vi "car_tcp.vi"() -> ()   [LabVIEW 2022 SP3]
uses:
  Control 1.ctl
  Control 2.ctl
  chicken.ctl
  plus_one.ctl
  game_over.ctl
  Control 4.ctl
  tree_control.ctl
panel:
  out "Boolean 12":T1
  in  "chicken":T2
  in  "tree 2":T3
  in  "tree":T3
  in  "tree 5":T3
  in  "tree 4":T3
  out "TOP":i16
  out "SCORE":i16
  in  "stop":bool
  in  "tree 3":T3
  out "Boolean 11":T4
  out "grass 5":T5
  out "grass 4":T5
  out "grass 3":T5
  out "grass 2":T5
  out "grass 1":T5
  out "easy?":bool
  in  "HARD":bool
  in  "EASY":bool
  out "car_x":i16
  out "Boolean 10":T6
  in  "v 10":dbl
  in  "v 9":dbl
  out "Boolean 9":T7
  in  "v 8":dbl
  out "Boolean 8":T6
  in  "v 7":dbl
  out "Boolean 7":T7
  out "Boolean 6":T6
  in  "v 6":dbl
  in  "v 5":dbl
  out "Boolean 5":T7
  in  "v 4":dbl
  out "Boolean 4":T6
  in  "v 3":dbl
  out "Boolean 3":T7
  in  "v 2":dbl
  in  "v":dbl
  out "Boolean 2":T6
  out "Boolean":T7
  # "SCORE"
  # "TOP"
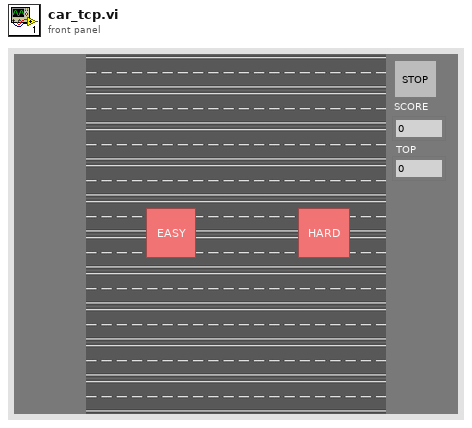
[diagram p1: front panel]
types:
  T1 = typedef "game_over.ctl" = bool
  T2 = typedef "chicken.ctl" = bool
  T3 = typedef "tree_control.ctl" = bool
  T4 = typedef "plus_one.ctl" = bool
  T5 = typedef "Control 4.ctl" = bool
  T6 = typedef "Control 2.ctl" = bool
  T7 = typedef "Control 1.ctl" = bool
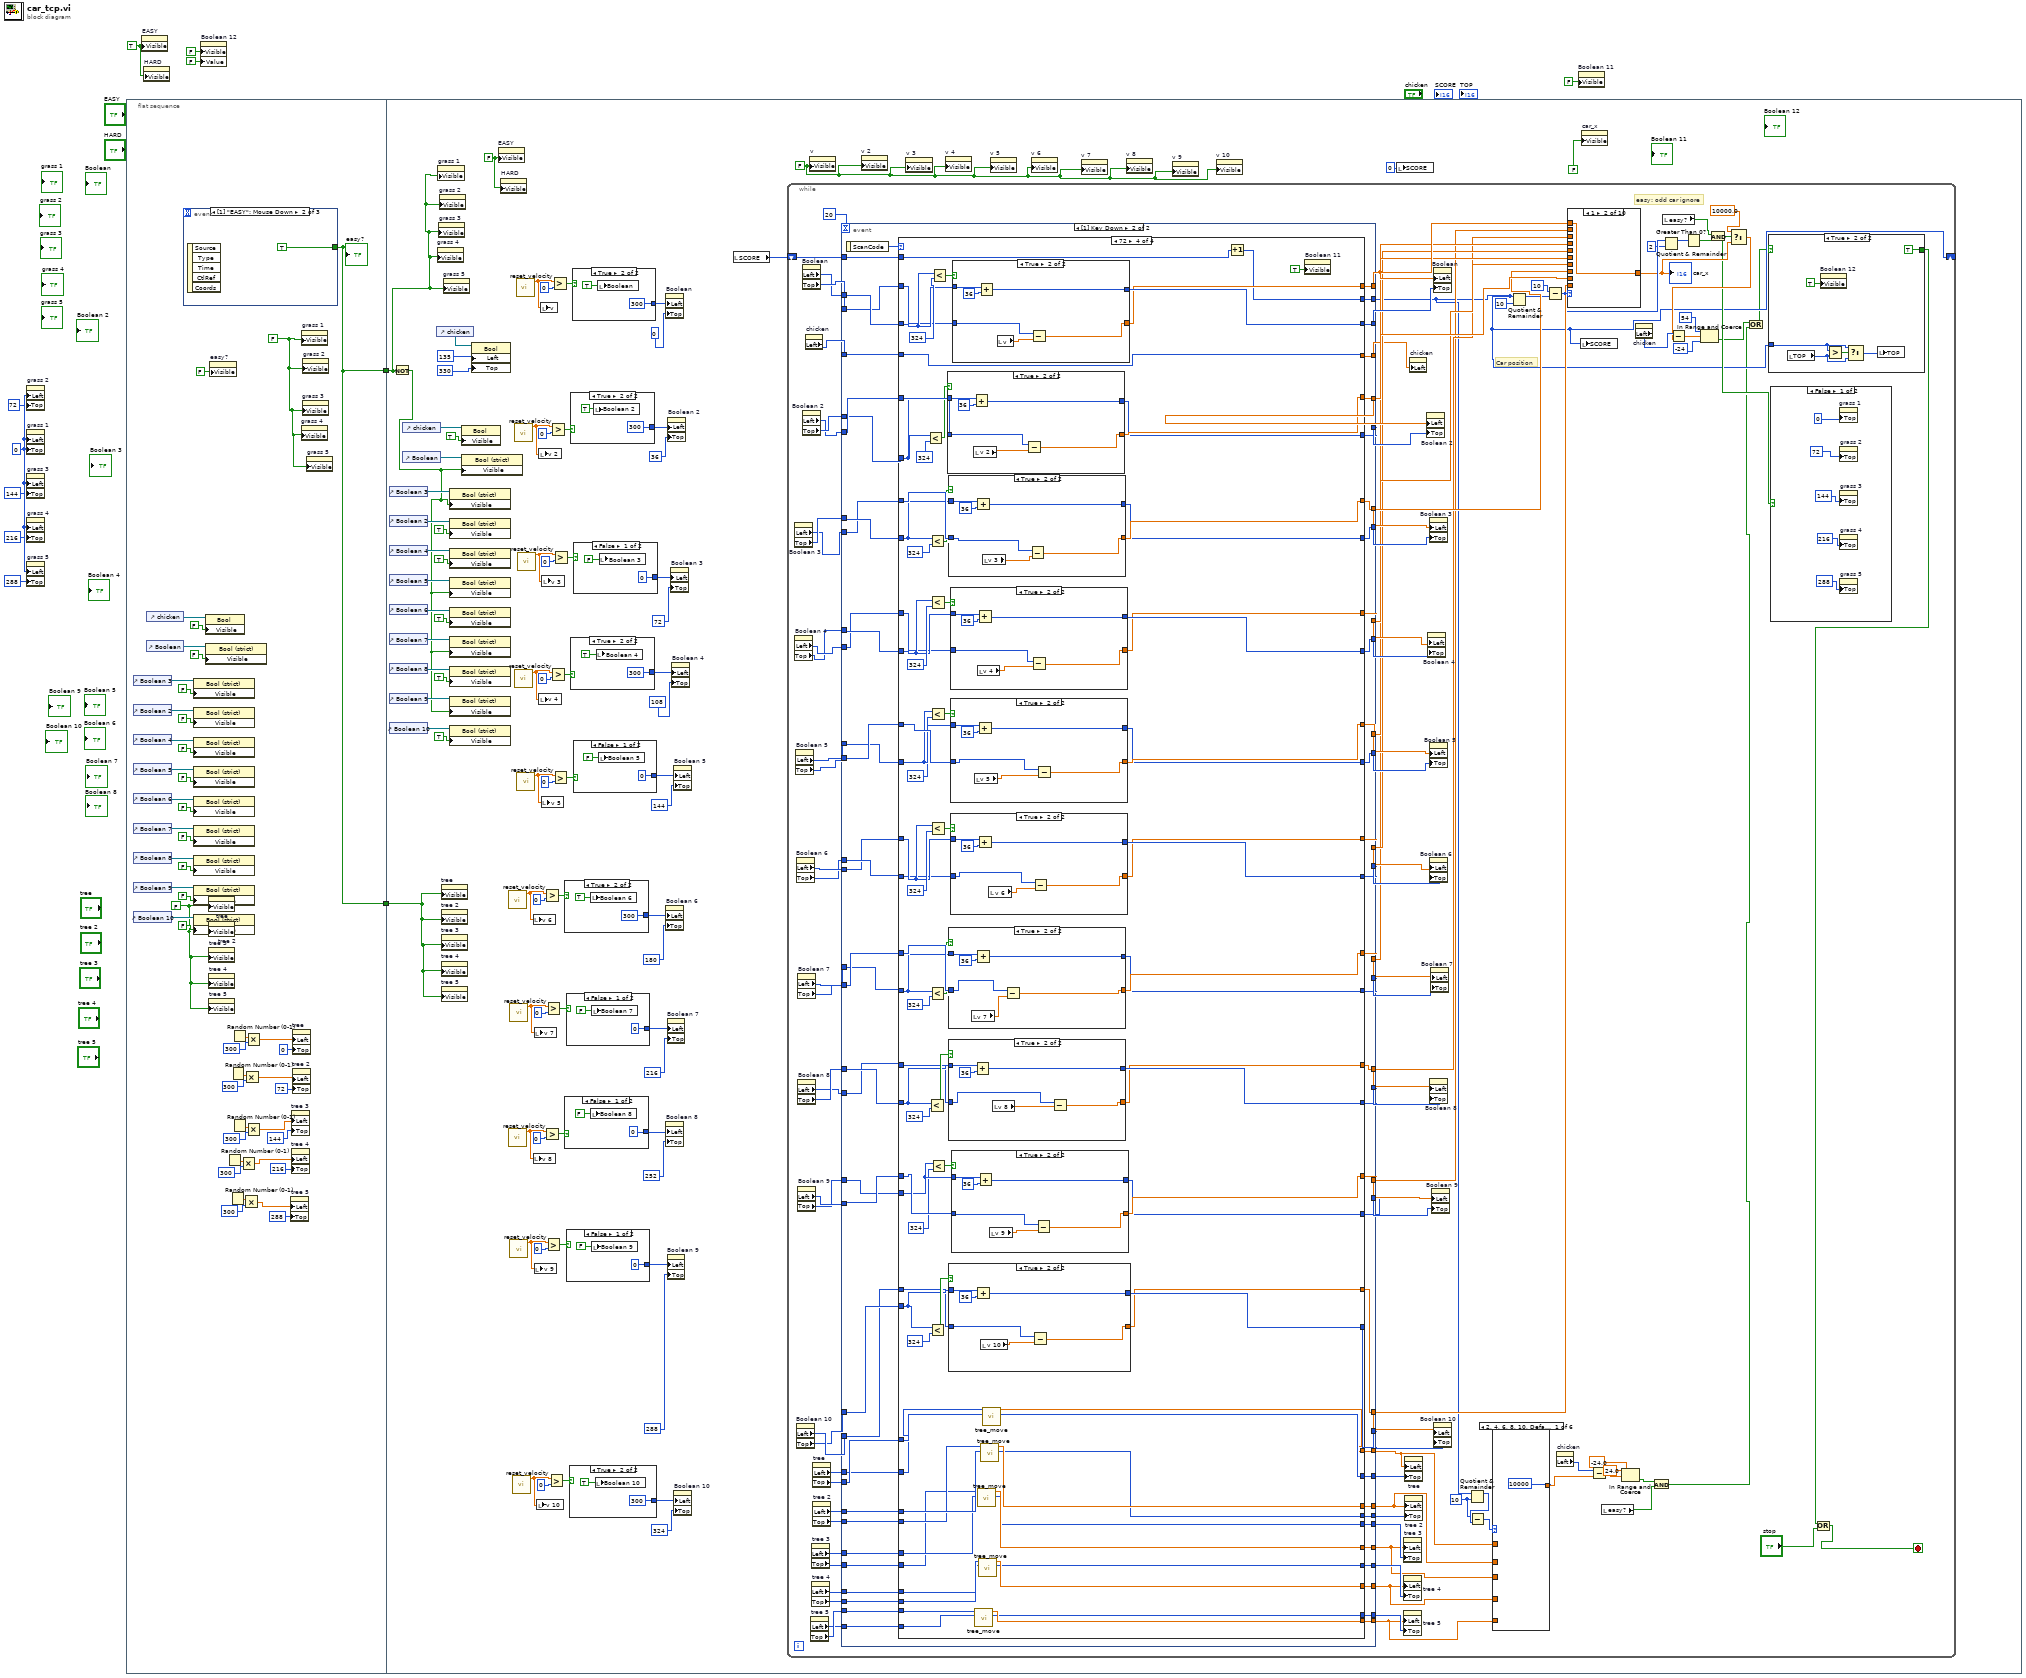
[diagram p0: block diagram]
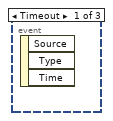
[diagram p2: hidden frame]
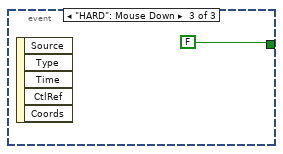
[diagram p3: hidden frame]
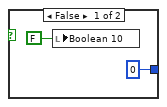
[diagram p4: hidden frame]
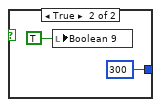
[diagram p5: hidden frame]
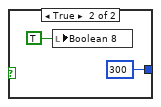
[diagram p6: hidden frame]
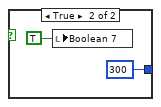
[diagram p7: hidden frame]
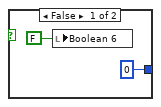
[diagram p8: hidden frame]
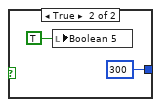
[diagram p9: hidden frame]
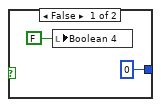
[diagram p10: hidden frame]
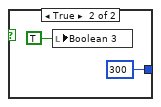
[diagram p11: hidden frame]
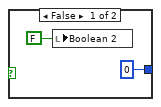
[diagram p12: hidden frame]
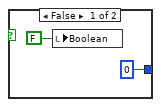
[diagram p13: hidden frame]
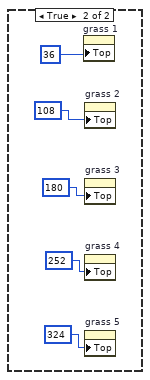
[diagram p19: hidden frame]
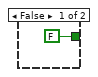
[diagram p20: hidden frame]
diagram:
  w6 = 0
  w8 = TRUE ("Visible")
  n1 = property on="grass 2" class="Bool"("Left"=w6, "Top"=72) -> ()  [unwired: 2 in, 2 out]
  n2 = property on="grass 1" class="Bool"("Left"=w6, "Top"=w6) -> ()  [unwired: 2 in, 2 out]
  n3 = property on="grass 3" class="Bool"("Left"=w6, "Top"=144) -> ()  [unwired: 2 in, 2 out]
  n4 = property on="grass 4" class="Bool"("Left"=w6, "Top"=216) -> ()  [unwired: 2 in, 2 out]
  n5 = property on="grass 5" class="Bool"("Left"=w6, "Top"=288) -> ()  [unwired: 2 in, 2 out]
  n6 = flat-sequence {
    tunnel: [w32] -> w7
    tunnel: [w32] -> w1
    tunnel: w7 -> [w62]
    tunnel: w1 -> [w60]
    frame #0 {
      w33 = FALSE
      w34 = FALSE ("Visible")
      n7 = control-ref of="Boolean 3"() -> (w44:refnum<vi>)
      n8 = control-ref of="Boolean 2"() -> (w43:refnum<vi>)
      n9 = control-ref of="Boolean 4"() -> (w42:refnum<vi>)
      n10 = control-ref of="Boolean 5"() -> (w41:refnum<vi>)
      n11 = control-ref of="Boolean 6"() -> (w40:refnum<vi>)
      n12 = control-ref of="Boolean 7"() -> (w39:refnum<vi>)
      n13 = control-ref of="Boolean 8"() -> (w38:refnum<vi>)
      n14 = control-ref of="Boolean 9"() -> (w37:refnum<vi>)
      n15 = control-ref of="Boolean 10"() -> (w35:refnum<vi>)
      n16 = control-ref of="chicken"() -> (w56:refnum<vi>)
      n17 = control-ref of="Boolean"() -> (w45:refnum<vi>)
      n18 = event shown="[1] \"EASY\": Mouse Down" {
        selector: _ -> [_ _ _]
        dyn-events: _ -> [_ _ _]
        timeout: _ -> [_ _ _]
        tunnel: [_ TRUE FALSE] -> w32
        event Timeout {
          n19 = event-data() -> ()  [unwired: 1 in, 3 out]
        }
        event "EASY": Mouse Down {
          n20 = event-data() -> ()  [unwired: 1 in, 5 out]
        }
        event "HARD": Mouse Down {
          n21 = event-data() -> ()  [unwired: 1 in, 5 out]
        }
      }
      "easy?" <- w32
      n22 = property class="Bool (strict)"(reference=w44, "Visible"=FALSE) -> ()  [unwired: 1 in, 2 out]
      n23 = property class="Bool (strict)"(reference=w43, "Visible"=FALSE) -> ()  [unwired: 1 in, 2 out]
      n24 = property class="Bool (strict)"(reference=w42, "Visible"=FALSE) -> ()  [unwired: 1 in, 2 out]
      n25 = property class="Bool (strict)"(reference=w41, "Visible"=FALSE) -> ()  [unwired: 1 in, 2 out]
      n26 = property class="Bool (strict)"(reference=w40, "Visible"=FALSE) -> ()  [unwired: 1 in, 2 out]
      n27 = property class="Bool (strict)"(reference=w39, "Visible"=FALSE) -> ()  [unwired: 1 in, 2 out]
      n28 = property class="Bool (strict)"(reference=w38, "Visible"=FALSE) -> ()  [unwired: 1 in, 2 out]
      n29 = property class="Bool (strict)"(reference=w37, "Visible"=FALSE) -> ()  [unwired: 1 in, 2 out]
      n30 = property class="Bool (strict)"(reference=w35, "Visible"=FALSE) -> ()  [unwired: 1 in, 2 out]
      n31 = property class="Bool"(reference=w56, "Visible"=FALSE) -> ()  [unwired: 1 in, 2 out]
      n32 = property class="Bool (strict)"(reference=w45, "Visible"=FALSE) -> ()  [unwired: 1 in, 2 out]
      n33 = property on="tree" class="Bool"("Visible"=w33) -> ()  [unwired: 2 in, 2 out]
      n34 = property on="tree 2" class="Bool"("Visible"=w33) -> ()  [unwired: 2 in, 2 out]
      n35 = property on="tree 3" class="Bool"("Visible"=w33) -> ()  [unwired: 2 in, 2 out]
      n36 = property on="tree 4" class="Bool"("Visible"=w33) -> ()  [unwired: 2 in, 2 out]
      n37 = property on="tree 5" class="Bool"("Visible"=w33) -> ()  [unwired: 2 in, 2 out]
      n38 = property on="easy?" class="Bool (strict)"("Visible"=FALSE) -> ()  [unwired: 2 in, 2 out]
      n39 = Random Number (0-1)() -> (number: 0 to 1=w23:dbl)
      n40 = Random Number (0-1)() -> (number: 0 to 1=w22:dbl)
      n41 = Random Number (0-1)() -> (number: 0 to 1=w27:dbl)
      n42 = Random Number (0-1)() -> (number: 0 to 1=w31:dbl)
      n43 = Random Number (0-1)() -> (number: 0 to 1=w26:dbl)
      n44 = Multiply(x=w23, y=300) -> (x*y=w18:dbl)
      n45 = Multiply(x=w22, y=300) -> (x*y=w17:dbl)
      n46 = Multiply(x=w27, y=300) -> (x*y=w20:dbl)
      n47 = Multiply(x=w31, y=300) -> (x*y=w29:dbl)
      n48 = Multiply(x=w26, y=300) -> (x*y=w19:dbl)
      n49 = property on="tree 5" class="Bool"("Left"=w17, "Top"=288 ("Position:Top")) -> ()  [unwired: 2 in, 2 out]
      n50 = property on="tree 3" class="Bool"("Left"=w19, "Top"=144 ("Position:Top")) -> ()  [unwired: 2 in, 2 out]
      n51 = property on="tree 4" class="Bool"("Left"=w18, "Top"=216 ("Position:Top")) -> ()  [unwired: 2 in, 2 out]
      n52 = property on="tree" class="Bool"("Left"=w29, "Top"=0 ("Position:Top")) -> ()  [unwired: 2 in, 2 out]
      n53 = property on="tree 2" class="Bool"("Left"=w20, "Top"=72 ("Position:Top")) -> ()  [unwired: 2 in, 2 out]
      n54 = property on="grass 4" class="Bool"("Visible"=w34) -> ()  [unwired: 2 in, 2 out]
      n55 = property on="grass 1" class="Bool"("Visible"=w34) -> ()  [unwired: 2 in, 2 out]
      n56 = property on="grass 3" class="Bool"("Visible"=w34) -> ()  [unwired: 2 in, 2 out]
      n57 = property on="grass 2" class="Bool"("Visible"=w34) -> ()  [unwired: 2 in, 2 out]
      n58 = property on="grass 5" class="Bool"("Visible"=w34) -> ()  [unwired: 2 in, 2 out]
    }
    frame #1 {
      w81 = FALSE ("Visible")
      w96 = FALSE ("Visible")
      n59 = control-ref of="Boolean 3"() -> (w71:refnum<vi>)
      n60 = control-ref of="Boolean 2"() -> (w72:refnum<vi>)
      n61 = control-ref of="Boolean 4"() -> (w73:refnum<vi>)
      n62 = control-ref of="Boolean 5"() -> (w74:refnum<vi>)
      n63 = control-ref of="Boolean 6"() -> (w75:refnum<vi>)
      n64 = control-ref of="Boolean 7"() -> (w76:refnum<vi>)
      n65 = control-ref of="Boolean 8"() -> (w77:refnum<vi>)
      n66 = control-ref of="Boolean 9"() -> (w78:refnum<vi>)
      n67 = control-ref of="Boolean 10"() -> (w80:refnum<vi>)
      n68 = Not(x=w62) -> (.not. x?=w63:bool)
      n69 = control-ref of="chicken"() -> (w64:refnum<vi>)
      n70 = control-ref of="Boolean"() -> (w70:refnum<vi>)
      n71 = control-ref of="chicken"() -> (w86:refnum<vi>)
      n72 = property on="grass 4" class="Bool"("Visible"=w62) -> ()  [unwired: 2 in, 2 out]
      n73 = property on="grass 1" class="Bool"("Visible"=w62) -> ()  [unwired: 2 in, 2 out]
      n74 = property on="grass 3" class="Bool"("Visible"=w62) -> ()  [unwired: 2 in, 2 out]
      n75 = property on="grass 2" class="Bool"("Visible"=w62) -> ()  [unwired: 2 in, 2 out]
      n76 = property on="tree" class="Bool"("Visible"=w60) -> ()  [unwired: 2 in, 2 out]
      n77 = property on="tree 2" class="Bool"("Visible"=w60) -> ()  [unwired: 2 in, 2 out]
      n78 = property on="tree 3" class="Bool"("Visible"=w60) -> ()  [unwired: 2 in, 2 out]
      n79 = property on="tree 4" class="Bool"("Visible"=w60) -> ()  [unwired: 2 in, 2 out]
      n80 = property on="tree 5" class="Bool"("Visible"=w60) -> ()  [unwired: 2 in, 2 out]
      n81 = property on="grass 5" class="Bool"("Visible"=w62) -> ()  [unwired: 2 in, 2 out]
      n82 = property class="Bool (strict)"(reference=w71, "Visible"=w63) -> ()  [unwired: 1 in, 2 out]
      n83 = property class="Bool (strict)"(reference=w72, "Visible"=TRUE) -> ()  [unwired: 1 in, 2 out]
      n84 = property class="Bool (strict)"(reference=w73, "Visible"=TRUE) -> ()  [unwired: 1 in, 2 out]
      n85 = property class="Bool (strict)"(reference=w74, "Visible"=w63) -> ()  [unwired: 1 in, 2 out]
      n86 = property class="Bool (strict)"(reference=w75, "Visible"=TRUE) -> ()  [unwired: 1 in, 2 out]
      n87 = property class="Bool (strict)"(reference=w76, "Visible"=w63) -> ()  [unwired: 1 in, 2 out]
      n88 = property class="Bool (strict)"(reference=w77, "Visible"=TRUE) -> ()  [unwired: 1 in, 2 out]
      n89 = property class="Bool (strict)"(reference=w78, "Visible"=w63) -> ()  [unwired: 1 in, 2 out]
      n90 = property class="Bool (strict)"(reference=w80, "Visible"=TRUE) -> ()  [unwired: 1 in, 2 out]
      n91 = property class="Bool"(reference=w64, "Visible"=TRUE) -> ()  [unwired: 1 in, 2 out]
      n92 = property class="Bool (strict)"(reference=w70, "Visible"=w63) -> ()  [unwired: 1 in, 2 out]
      n93 = property on="Property Node" class="Bool"(reference=w86, "Left"=135 ("Position:Left"), "Top"=330 ("Position:Top")) -> ()  [unwired: 1 in, 2 out]
      n94 = property on="EASY" class="Bool"("Visible"=w81) -> ()  [unwired: 2 in, 2 out]
      n95 = property on="HARD" class="Bool"("Visible"=w81) -> ()  [unwired: 2 in, 2 out]
      n96 = call "reset_velocity.vi"() -> ("Numeric"=w91:dbl)  [unwired: 11 in]
      n97 = call "reset_velocity.vi"() -> ("Numeric"=w89:dbl)  [unwired: 11 in]
      n98 = call "reset_velocity.vi"() -> ("Numeric"=w90:dbl)  [unwired: 11 in]
      n99 = call "reset_velocity.vi"() -> ("Numeric"=w88:dbl)  [unwired: 11 in]
      n100 = call "reset_velocity.vi"() -> ("Numeric"=w87:dbl)  [unwired: 11 in]
      n101 = call "reset_velocity.vi"() -> ("Numeric"=w95:dbl)  [unwired: 11 in]
      n102 = call "reset_velocity.vi"() -> ("Numeric"=w93:dbl)  [unwired: 11 in]
      n103 = call "reset_velocity.vi"() -> ("Numeric"=w137:dbl)  [unwired: 11 in]
      n104 = call "reset_velocity.vi"() -> ("Numeric"=w92:dbl)  [unwired: 11 in]
      n105 = call "reset_velocity.vi"() -> ("Numeric"=w94:dbl)  [unwired: 11 in]
      n106 = local write "v 6"(w91) -> ()
      n107 = local write "v 8"(w89) -> ()
      n108 = local write "v 7"(w90) -> ()
      n109 = local write "v 9"(w88) -> ()
      n110 = local write "v 10"(w87) -> ()
      n111 = local write "v 2"(w95) -> ()
      n112 = local write "v 4"(w93) -> ()
      n113 = local write "v"(w137) -> ()
      n114 = local write "v 5"(w92) -> ()
      n115 = local write "v 3"(w94) -> ()
      n116 = Greater?(x=w91, y=0) -> (0:w116:bool)
      n117 = Greater?(x=w89, y=0) -> (0:w108:bool)
      n118 = Greater?(x=w90, y=0) -> (0:w111:bool)
      n119 = Greater?(x=w88, y=0) -> (0:w103:bool)
      n120 = Greater?(x=w87, y=0) -> (0:w100:bool)
      n121 = Greater?(x=w95, y=0) -> (0:w132:bool)
      n122 = Greater?(x=w93, y=0) -> (0:w124:bool)
      n123 = Greater?(x=w137, y=0) -> (0:w135:bool)
      n124 = Greater?(x=w92, y=0) -> (0:w119:bool)
      n125 = Greater?(x=w94, y=0) -> (0:w127:bool)
      n126 = case shown="True" w116 {
        tunnel: [0 300] -> w114
        frame False {
          n127 = local write "Boolean 6"(FALSE) -> ()
        }
        frame True {
          n128 = local write "Boolean 6"(TRUE) -> ()
        }
      }
      n129 = case shown="False" w108 {
        tunnel: [0 300] -> w106
        frame False {
          n130 = local write "Boolean 8"(FALSE) -> ()
        }
        frame True {
          n131 = local write "Boolean 8"(TRUE) -> ()
        }
      }
      n132 = case shown="False" w111 {
        tunnel: [0 300] -> w110
        frame False {
          n133 = local write "Boolean 7"(FALSE) -> ()
        }
        frame True {
          n134 = local write "Boolean 7"(TRUE) -> ()
        }
      }
      n135 = case shown="False" w103 {
        tunnel: [0 300] -> w102
        frame False {
          n136 = local write "Boolean 9"(FALSE) -> ()
        }
        frame True {
          n137 = local write "Boolean 9"(TRUE) -> ()
        }
      }
      n138 = case shown="True" w100 {
        tunnel: [0 300] -> w98
        frame False {
          n139 = local write "Boolean 10"(FALSE) -> ()
        }
        frame True {
          n140 = local write "Boolean 10"(TRUE) -> ()
        }
      }
      n141 = case shown="True" w132 {
        tunnel: [0 300] -> w130
        frame False {
          n142 = local write "Boolean 2"(FALSE) -> ()
        }
        frame True {
          n143 = local write "Boolean 2"(TRUE) -> ()
        }
      }
      n144 = case shown="True" w124 {
        tunnel: [0 300] -> w122
        frame False {
          n145 = local write "Boolean 4"(FALSE) -> ()
        }
        frame True {
          n146 = local write "Boolean 4"(TRUE) -> ()
        }
      }
      n147 = case shown="True" w135 {
        tunnel: [0 300] -> w134
        frame False {
          n148 = local write "Boolean"(FALSE) -> ()
        }
        frame True {
          n149 = local write "Boolean"(TRUE) -> ()
        }
      }
      n150 = case shown="False" w119 {
        tunnel: [0 300] -> w118
        frame False {
          n151 = local write "Boolean 5"(FALSE) -> ()
        }
        frame True {
          n152 = local write "Boolean 5"(TRUE) -> ()
        }
      }
      n153 = case shown="False" w127 {
        tunnel: [0 300] -> w125
        frame False {
          n154 = local write "Boolean 3"(FALSE) -> ()
        }
        frame True {
          n155 = local write "Boolean 3"(TRUE) -> ()
        }
      }
      n156 = property on="Boolean" class="Bool (strict)"("Left"=w134, "Top"=0) -> ()  [unwired: 2 in, 2 out]
      n157 = property on="Boolean 6" class="Bool (strict)"("Left"=w114, "Top"=180) -> ()  [unwired: 2 in, 2 out]
      n158 = property on="Boolean 8" class="Bool (strict)"("Left"=w106, "Top"=252) -> ()  [unwired: 2 in, 2 out]
      n159 = property on="Boolean 7" class="Bool (strict)"("Left"=w110, "Top"=216) -> ()  [unwired: 2 in, 2 out]
      n160 = property on="Boolean 9" class="Bool (strict)"("Left"=w102, "Top"=288) -> ()  [unwired: 2 in, 2 out]
      n161 = property on="Boolean 2" class="Bool (strict)"("Left"=w130, "Top"=36) -> ()  [unwired: 2 in, 2 out]
      n162 = property on="Boolean 3" class="Bool (strict)"("Left"=w125, "Top"=72) -> ()  [unwired: 2 in, 2 out]
      n163 = property on="Boolean 4" class="Bool (strict)"("Left"=w122, "Top"=108) -> ()  [unwired: 2 in, 2 out]
      n164 = property on="Boolean 5" class="Bool (strict)"("Left"=w118, "Top"=144) -> ()  [unwired: 2 in, 2 out]
      n165 = property on="Boolean 10" class="Bool (strict)"("Left"=w98, "Top"=324) -> ()  [unwired: 2 in, 2 out]
      n166 = local read "SCORE"() -> (w61:i16)
      n167 = while {
        shift-right: [w196] -> _
        shift-left: w61 -> [w212]
        stop <- w230 stop-if-true
        w194 = i16 10 ("y")
        # "easy: odd car ignore"
        # "Car position"
        n168 = property on="Boolean 3" class="Bool (strict)"() -> ("Left"=w266:i32, "Top"=w267:i32)  [unwired: 2 in, 2 out]
        n169 = property on="Boolean 4" class="Bool (strict)"() -> ("Left"=w264:i32, "Top"=w263:i32)  [unwired: 2 in, 2 out]
        n170 = property on="Boolean 5" class="Bool (strict)"() -> ("Left"=w253:i32, "Top"=w261:i32)  [unwired: 2 in, 2 out]
        n171 = property on="Boolean 6" class="Bool (strict)"() -> ("Left"=w259:i32, "Top"=w258:i32)  [unwired: 2 in, 2 out]
        n172 = property on="Boolean 10" class="Bool (strict)"() -> ("Left"=w246:i32, "Top"=w245:i32)  [unwired: 2 in, 2 out]
        n173 = property on="Boolean 7" class="Bool (strict)"() -> ("Left"=w252:i32, "Top"=w256:i32)  [unwired: 2 in, 2 out]
        n174 = property on="Boolean 8" class="Bool (strict)"() -> ("Left"=w251:i32, "Top"=w254:i32)  [unwired: 2 in, 2 out]
        n175 = property on="Boolean 9" class="Bool (strict)"() -> ("Left"=w249:i32, "Top"=w248:i32)  [unwired: 2 in, 2 out]
        n176 = property on="Boolean" class="Bool (strict)"() -> ("Left"=w272:i32, "Top"=w273:i32)  [unwired: 2 in, 2 out]
        n177 = property on="Boolean 2" class="Bool (strict)"() -> ("Left"=w270:i32, "Top"=w271:i32)  [unwired: 2 in, 2 out]
        n178 = property on="chicken" class="Bool"() -> ("Left"=w216:i32)  [unwired: 2 in, 2 out]
        n179 = property on="tree 5" class="Bool"() -> ("Left"=w201:i32, "Top"=w202:i32)  [unwired: 2 in, 2 out]
        n180 = property on="tree 3" class="Bool"() -> ("Left"=w206:i32, "Top"=w205:i32)  [unwired: 2 in, 2 out]
        n181 = property on="tree 4" class="Bool"() -> ("Left"=w203:i32, "Top"=w204:i32)  [unwired: 2 in, 2 out]
        n182 = property on="tree" class="Bool"() -> ("Left"=w210:i32, "Top"=w211:i32)  [unwired: 2 in, 2 out]
        n183 = property on="tree 2" class="Bool"() -> ("Left"=w208:i32, "Top"=w207:i32)  [unwired: 2 in, 2 out]
        n184 = event shown="[1] Key Down" {
          selector: _ -> [_ _]
          dyn-events: _ -> [_ _]
          timeout: 20 -> [_ _]
          tunnel: [w393 w554] -> w268
          tunnel: [w395 w552] -> w242
          tunnel: w272 -> [w394 w551]
          tunnel: w273 -> [w393 w553]
          tunnel: [w392 w547] -> w269
          tunnel: [w390 w548] -> w241
          tunnel: w270 -> [w391 w550]
          tunnel: w271 -> [w392 w549]
          tunnel: [w384 w543] -> w265
          tunnel: [w382 w544] -> w240
          tunnel: w266 -> [w383 w545]
          tunnel: w267 -> [w384 w546]
          tunnel: [w369 w539] -> w262
          tunnel: [w371 w540] -> w239
          tunnel: w264 -> [w370 w541]
          tunnel: w263 -> [w369 w542]
          tunnel: [w368 w536] -> w260
          tunnel: [w366 w535] -> w238
          tunnel: w253 -> [w367 w538]
          tunnel: w261 -> [w368 w537]
          tunnel: [w353 w531] -> w257
          tunnel: [w355 w532] -> w237
          tunnel: w259 -> [w354 w533]
          tunnel: w258 -> [w353 w534]
          tunnel: [w352 w527] -> w255
          tunnel: [w350 w528] -> w236
          tunnel: w252 -> [w351 w530]
          tunnel: w256 -> [w352 w529]
          tunnel: [w337 w523] -> w250
          tunnel: [w339 w524] -> w235
          tunnel: w251 -> [w338 w525]
          tunnel: w254 -> [w337 w526]
          tunnel: [w336 w519] -> w247
          tunnel: [w334 w520] -> w234
          tunnel: w249 -> [w335 w522]
          tunnel: w248 -> [w336 w521]
          tunnel: [w321 w515] -> w244
          tunnel: [w323 w516] -> w233
          tunnel: w246 -> [w322 w517]
          tunnel: w245 -> [w321 w518]
          tunnel: w216 -> [w319 w514]
          tunnel: [w319 w513] -> w215
          tunnel: w212 -> [w318 w512]
          tunnel: [w318 w511] -> w196
          tunnel: w211 -> [w316 w510]
          tunnel: w210 -> [w317 w509]
          tunnel: [w316 w508] -> w209
          tunnel: [w317 w507] -> w192
          tunnel: w208 -> [w315 w506]
          tunnel: w207 -> [w314 w505]
          tunnel: w206 -> [w313 w504]
          tunnel: w205 -> [w312 w503]
          tunnel: w204 -> [w310 w502]
          tunnel: w203 -> [w311 w501]
          tunnel: w202 -> [w309 w500]
          tunnel: w201 -> [w308 w499]
          tunnel: [w315 w498] -> w191
          tunnel: [w314 w497] -> w200
          tunnel: [w313 w496] -> w190
          tunnel: [w312 w495] -> w199
          tunnel: [w311 w494] -> w189
          tunnel: [w310 w493] -> w198
          tunnel: [w308 w492] -> w188
          tunnel: [w309 w491] -> w197
          event Timeout {
            n185 = event-data() -> ()  [unwired: 1 in, 1 out]
            n186 = Greater Or Equal?(x=w394, y=-62) -> (x >= y?=w399:bool)
            n187 = Less Or Equal?(x=w394, y=300) -> (x <= y?=w400:bool)
            n188 = Greater Or Equal?(x=w391, y=-62) -> (x >= y?=w386:bool)
            n189 = Greater Or Equal?(x=w367, y=-62) -> (x >= y?=w362:bool)
            n190 = Less Or Equal?(x=w391, y=300) -> (x <= y?=w385:bool)
            n191 = Greater Or Equal?(x=w383, y=-62) -> (x >= y?=w378:bool)
            n192 = Greater Or Equal?(x=w370, y=-62) -> (x >= y?=w375:bool)
            n193 = Less Or Equal?(x=w367, y=300) -> (x <= y?=w361:bool)
            n194 = Less Or Equal?(x=w383, y=300) -> (x <= y?=w377:bool)
            n195 = Less Or Equal?(x=w370, y=300) -> (x <= y?=w376:bool)
            n196 = Greater Or Equal?(x=w354, y=-62) -> (x >= y?=w359:bool)
            n197 = Less Or Equal?(x=w354, y=300) -> (x <= y?=w360:bool)
            n198 = Greater Or Equal?(x=w351, y=-62) -> (x >= y?=w346:bool)
            n199 = Greater Or Equal?(x=w338, y=-62) -> (x >= y?=w343:bool)
            n200 = Less Or Equal?(x=w351, y=300) -> (x <= y?=w345:bool)
            n201 = Less Or Equal?(x=w338, y=300) -> (x <= y?=w344:bool)
            n202 = Greater Or Equal?(x=w335, y=-62) -> (x >= y?=w330:bool)
            n203 = Less Or Equal?(x=w335, y=300) -> (x <= y?=w329:bool)
            n204 = Greater Or Equal?(x=w322, y=-62) -> (x >= y?=w327:bool)
            n205 = Less Or Equal?(x=w322, y=300) -> (x <= y?=w328:bool)
            n206 = And(x=w399, y=w400) -> (x .and. y?=w398:bool)
            n207 = And(x=w386, y=w385) -> (x .and. y?=w387:bool)
            n208 = And(x=w362, y=w361) -> (x .and. y?=w363:bool)
            n209 = And(x=w378, y=w377) -> (x .and. y?=w379:bool)
            n210 = And(x=w375, y=w376) -> (x .and. y?=w374:bool)
            n211 = And(x=w359, y=w360) -> (x .and. y?=w358:bool)
            n212 = And(x=w346, y=w345) -> (x .and. y?=w347:bool)
            n213 = And(x=w343, y=w344) -> (x .and. y?=w342:bool)
            n214 = And(x=w330, y=w329) -> (x .and. y?=w331:bool)
            n215 = And(x=w327, y=w328) -> (x .and. y?=w326:bool)
            n216 = case shown="True" w398 {
              tunnel: [w482 w489] -> w395
              tunnel: w394 -> [_ w488]
              frame False {
                n217 = local read "v"() -> (w485:dbl)
                n218 = Greater?(x=w485, y=0) -> (0:w483:bool)
                n219 = case shown="False" w483 {
                  tunnel: [0 300] -> w482
                  frame False {
                  }
                  frame True {
                  }
                }
              }
              frame True {
                n220 = Subtract(x=w488, y="v") -> (x-y=w489:dbl)
              }
            }
            n221 = case shown="True" w387 {
              tunnel: [w473 w480] -> w390
              tunnel: w391 -> [_ w479]
              frame False {
                n222 = local read "v 2"() -> (w476:dbl)
                n223 = Greater?(x=w476, y=0) -> (0:w474:bool)
                n224 = case shown="False" w474 {
                  tunnel: [0 300] -> w473
                  frame False {
                  }
                  frame True {
                  }
                }
              }
              frame True {
                n225 = Subtract(x=w479, y="v 2") -> (x-y=w480:dbl)
              }
            }
            n226 = case shown="True" w363 {
              tunnel: [w446 w453] -> w366
              tunnel: w367 -> [_ w452]
              frame False {
                n227 = local read "v 5"() -> (w449:dbl)
                n228 = Greater?(x=w449, y=0) -> (0:w447:bool)
                n229 = case shown="False" w447 {
                  tunnel: [0 300] -> w446
                  frame False {
                  }
                  frame True {
                  }
                }
              }
              frame True {
                n230 = Subtract(x=w452, y="v 5") -> (x-y=w453:dbl)
              }
            }
            n231 = case shown="True" w379 {
              tunnel: [w464 w471] -> w382
              tunnel: w383 -> [_ w470]
              frame False {
                n232 = local read "v 3"() -> (w467:dbl)
                n233 = Greater?(x=w467, y=0) -> (0:w465:bool)
                n234 = case shown="False" w465 {
                  tunnel: [0 300] -> w464
                  frame False {
                  }
                  frame True {
                  }
                }
              }
              frame True {
                n235 = Subtract(x=w470, y="v 3") -> (x-y=w471:dbl)
              }
            }
            n236 = case shown="True" w374 {
              tunnel: [w455 w462] -> w371
              tunnel: w370 -> [_ w461]
              frame False {
                n237 = local read "v 4"() -> (w458:dbl)
                n238 = Greater?(x=w458, y=0) -> (0:w456:bool)
                n239 = case shown="False" w456 {
                  tunnel: [0 300] -> w455
                  frame False {
                  }
                  frame True {
                  }
                }
              }
              frame True {
                n240 = Subtract(x=w461, y="v 4") -> (x-y=w462:dbl)
              }
            }
            n241 = case shown="True" w358 {
              tunnel: [w437 w444] -> w355
              tunnel: w354 -> [_ w443]
              frame False {
                n242 = local read "v 6"() -> (w440:dbl)
                n243 = Greater?(x=w440, y=0) -> (0:w438:bool)
                n244 = case shown="False" w438 {
                  tunnel: [0 300] -> w437
                  frame False {
                  }
                  frame True {
                  }
                }
              }
              frame True {
                n245 = Subtract(x=w443, y="v 6") -> (x-y=w444:dbl)
              }
            }
            n246 = case shown="True" w347 {
              tunnel: [w428 w435] -> w350
              tunnel: w351 -> [_ w434]
              frame False {
                n247 = local read "v 7"() -> (w431:dbl)
                n248 = Greater?(x=w431, y=0) -> (0:w429:bool)
                n249 = case shown="False" w429 {
                  tunnel: [0 300] -> w428
                  frame False {
                  }
                  frame True {
                  }
                }
              }
              frame True {
                n250 = Subtract(x=w434, y="v 7") -> (x-y=w435:dbl)
              }
            }
            n251 = case shown="True" w342 {
              tunnel: [w419 w426] -> w339
              tunnel: w338 -> [_ w425]
              frame False {
                n252 = local read "v 8"() -> (w422:dbl)
                n253 = Greater?(x=w422, y=0) -> (0:w420:bool)
                n254 = case shown="False" w420 {
                  tunnel: [0 300] -> w419
                  frame False {
                  }
                  frame True {
                  }
                }
              }
              frame True {
                n255 = Subtract(x=w425, y="v 8") -> (x-y=w426:dbl)
              }
            }
            n256 = case shown="True" w331 {
              tunnel: [w410 w417] -> w334
              tunnel: w335 -> [_ w416]
              frame False {
                n257 = local read "v 9"() -> (w413:dbl)
                n258 = Greater?(x=w413, y=0) -> (0:w411:bool)
                n259 = case shown="False" w411 {
                  tunnel: [0 300] -> w410
                  frame False {
                  }
                  frame True {
                  }
                }
              }
              frame True {
                n260 = Subtract(x=w416, y="v 9") -> (x-y=w417:dbl)
              }
            }
            n261 = case shown="True" w326 {
              tunnel: [w401 w408] -> w323
              tunnel: w322 -> [_ w407]
              frame False {
                n262 = local read "v 10"() -> (w404:dbl)
                n263 = Greater?(x=w404, y=0) -> (0:w402:bool)
                n264 = case shown="False" w402 {
                  tunnel: [0 300] -> w401
                  frame False {
                  }
                  frame True {
                  }
                }
              }
              frame True {
                n265 = Subtract(x=w407, y="v 10") -> (x-y=w408:dbl)
              }
            }
            n266 = property on="Boolean 11" class="Bool (strict)"("Visible"=FALSE) -> ()  [unwired: 2 in, 2 out]
          }
          event Key Down {
            n267 = event-data() -> ("ScanCode"=w555:i16)  [unwired: 1 in]
            n268 = case shown="72" w555 {
              tunnel: [w587 w617 w654 w744] -> w554
              tunnel: w553 -> [w587 w617 w654 w743]
              tunnel: [w586 w618 w655 w742] -> w552
              tunnel: w551 -> [w586 w618 w655 w741]
              tunnel: [w584 w599 w652 w737] -> w547
              tunnel: w549 -> [w584 w599 w652 w738]
              tunnel: [w585 w600 w653 w739] -> w548
              tunnel: w550 -> [w585 w600 w653 w740]
              tunnel: [w582 w616 w650 w731] -> w543
              tunnel: w546 -> [w582 w616 w650 w732]
              tunnel: [w583 w615 w651 w733] -> w544
              tunnel: w545 -> [w583 w615 w651 w734]
              tunnel: [w580 w613 w648 w726] -> w539
              tunnel: w542 -> [w580 w613 w648 w725]
              tunnel: [w581 w614 w649 w724] -> w540
              tunnel: w541 -> [w581 w614 w649 w723]
              tunnel: [w578 w611 w646 w719] -> w536
              tunnel: w537 -> [w578 w611 w646 w720]
              tunnel: [w579 w612 w647 w721] -> w535
              tunnel: w538 -> [w579 w612 w647 w722]
              tunnel: [w576 w609 w644 w714] -> w531
              tunnel: w534 -> [w576 w609 w644 w713]
              tunnel: [w577 w610 w645 w712] -> w532
              tunnel: w533 -> [w577 w610 w645 w711]
              tunnel: [w574 w607 w642 w707] -> w527
              tunnel: w529 -> [w574 w607 w642 w708]
              tunnel: [w575 w608 w643 w709] -> w528
              tunnel: w530 -> [w575 w608 w643 w710]
              tunnel: [w572 w605 w640 w702] -> w523
              tunnel: w526 -> [w572 w605 w640 w701]
              tunnel: [w573 w606 w641 w700] -> w524
              tunnel: w525 -> [w573 w606 w641 w699]
              tunnel: [w570 w603 w638 w695] -> w519
              tunnel: w521 -> [w570 w603 w638 w696]
              tunnel: [w571 w604 w639 w697] -> w520
              tunnel: w522 -> [w571 w604 w639 w698]
              tunnel: [w568 w601 w636 w690] -> w515
              tunnel: w518 -> [w568 w601 w636 w689]
              tunnel: [w569 w602 w637 w688] -> w516
              tunnel: w517 -> [w569 w602 w637 w687]
              tunnel: w514 -> [w567 w624 w659 w685]
              tunnel: [w567 w619 w656 w685] -> w513
              tunnel: w512 -> [w566 w598 w635 w684]
              tunnel: [w566 w598 w635 w683] -> w511
              tunnel: w510 -> [w565 w597 w634 w682]
              tunnel: w509 -> [w564 w596 w627 w681]
              tunnel: [w565 w597 w634 w680] -> w508
              tunnel: [w564 w596 w627 w679] -> w507
              tunnel: w506 -> [w563 w595 w633 w678]
              tunnel: w505 -> [w562 w594 w632 w677]
              tunnel: w504 -> [w561 w593 w631 w676]
              tunnel: w503 -> [w560 w592 w630 w675]
              tunnel: w502 -> [w558 w590 w628 w674]
              tunnel: w501 -> [w559 w591 w629 w673]
              tunnel: w500 -> [w557 w589 w625 w672]
              tunnel: w499 -> [w556 w588 w626 w671]
              tunnel: [w563 w595 w633 w670] -> w498
              tunnel: [w562 w594 w632 w669] -> w497
              tunnel: [w561 w593 w631 w668] -> w496
              tunnel: [w560 w592 w630 w667] -> w495
              tunnel: [w559 w591 w629 w666] -> w494
              tunnel: [w558 w590 w628 w665] -> w493
              tunnel: [w556 w588 w626 w664] -> w492
              tunnel: [w557 w589 w625 w663] -> w491
              frame 0, Default {
              }
              frame 75 {
                # "Left"
                n269 = Subtract(x=w624, y=20) -> (x-y=w620:i32)
                n270 = Less Than 0?(x=w620) -> (x < 0?=w622:bool)
                n271 = Select(t=0.0, s=w622, f=w620) -> (s? t:f=w619:dbl)
              }
              frame 77 {
                n272 = Add(x=w659, y=20) -> (x+y=w658:i32)
                n273 = Greater?(x=w658, y=270) -> (0:w661:bool)
                n274 = Select(t=270.0, s=w661, f=w658) -> (s? t:f=w656:dbl)
              }
              frame 72 {
                n275 = Less?(x=w738, y=324) -> (x < y?=w735:bool)
                n276 = Less?(x=w701, y=324) -> (x < y?=w704:bool)
                n277 = Less?(x=w732, y=324) -> (x < y?=w729:bool)
                n278 = Less?(x=w708, y=324) -> (x < y?=w705:bool)
                n279 = Less?(x=w689, y=324) -> (x < y?=w692:bool)
                n280 = Less?(x=w725, y=324) -> (x < y?=w728:bool)
                n281 = Less?(x=w720, y=324) -> (x < y?=w717:bool)
                n282 = Less?(x=w713, y=324) -> (x < y?=w716:bool)
                n283 = Less?(x=w696, y=324) -> (x < y?=w693:bool)
                n284 = Less?(x=w743, y=324) -> (x < y?=w746:bool)
                n285 = case shown="True" w735 {
                  tunnel: [0 w881] -> w737
                  tunnel: w738 -> [_ w880]
                  tunnel: [w867 w878] -> w739
                  tunnel: w740 -> [_ w877]
                  frame False {
                    n286 = call "reset_velocity.vi"() -> ("Numeric"=w870:dbl)  [unwired: 11 in]
                    n287 = local write "v 2"(w870) -> ()
                    n288 = Greater?(x=w870, y=0) -> (0:w872:bool)
                    n289 = case shown="False" w872 {
                      frame False {
                        n290 = local write "Boolean 2"(FALSE) -> ()
                      }
                      frame True {
                        n291 = local write "Boolean 2"(TRUE) -> ()
                      }
                    }
                    n292 = Random Number (0-1)() -> (number: 0 to 1=w869:dbl)
                    n293 = Multiply(x=w869, y=300) -> (x*y=w867:dbl)
                  }
                  frame True {
                    n294 = Add(x=w880, y=36) -> (x+y=w881:i32)
                    n295 = local read "v 2"() -> (w876:dbl)
                    n296 = Subtract(x=w877, y=w876) -> (x-y=w878:dbl)
                  }
                }
                n297 = case shown="True" w704 {
                  tunnel: [0 w791] -> w702
                  tunnel: w701 -> [_ w790]
                  tunnel: [w777 w787] -> w700
                  tunnel: w699 -> [_ w788]
                  frame False {
                    n298 = call "reset_velocity.vi"() -> ("Numeric"=w780:dbl)  [unwired: 11 in]
                    n299 = local write "v 8"(w780) -> ()
                    n300 = Greater?(x=w780, y=0) -> (0:w782:bool)
                    n301 = case shown="False" w782 {
                      frame False {
                        n302 = local write "Boolean 8"(FALSE) -> ()
                      }
                      frame True {
                        (unwired) 300
                        n303 = local write "Boolean 8"(TRUE) -> ()
                      }
                    }
                    n304 = Random Number (0-1)() -> (number: 0 to 1=w778:dbl)
                    n305 = Multiply(x=w778, y=300) -> (x*y=w777:dbl)
                  }
                  frame True {
                    n306 = Add(x=w790, y=36) -> (x+y=w791:i32)
                    n307 = local read "v 8"() -> (w786:dbl)
                    n308 = Subtract(x=w788, y=w786) -> (x-y=w787:dbl)
                  }
                }
                n309 = case shown="True" w729 {
                  tunnel: [0 w866] -> w731
                  tunnel: w732 -> [_ w865]
                  tunnel: [w852 w862] -> w733
                  tunnel: w734 -> [_ w863]
                  frame False {
                    n310 = call "reset_velocity.vi"() -> ("Numeric"=w855:dbl)  [unwired: 11 in]
                    n311 = local write "v 3"(w855) -> ()
                    n312 = Greater?(x=w855, y=0) -> (0:w857:bool)
                    n313 = case shown="True" w857 {
                      frame False {
                        (unwired) 0
                        n314 = local write "Boolean 3"(FALSE) -> ()
                      }
                      frame True {
                        n315 = local write "Boolean 3"(TRUE) -> ()
                      }
                    }
                    n316 = Random Number (0-1)() -> (number: 0 to 1=w854:dbl)
                    n317 = Multiply(x=w854, y=300) -> (x*y=w852:dbl)
                  }
                  frame True {
                    n318 = Add(x=w865, y=36) -> (x+y=w866:i32)
                    n319 = local read "v 3"() -> (w861:dbl)
                    n320 = Subtract(x=w863, y=w861) -> (x-y=w862:dbl)
                  }
                }
                n321 = case shown="True" w705 {
                  tunnel: [0 w806] -> w707
                  tunnel: w708 -> [_ w805]
                  tunnel: [w792 w802] -> w709
                  tunnel: w710 -> [_ w803]
                  frame False {
                    n322 = call "reset_velocity.vi"() -> ("Numeric"=w795:dbl)  [unwired: 11 in]
                    n323 = local write "v 7"(w795) -> ()
                    n324 = Greater?(x=w795, y=0) -> (0:w797:bool)
                    n325 = case shown="True" w797 {
                      frame False {
                        (unwired) 0
                        n326 = local write "Boolean 7"(FALSE) -> ()
                      }
                      frame True {
                        n327 = local write "Boolean 7"(TRUE) -> ()
                      }
                    }
                    n328 = Random Number (0-1)() -> (number: 0 to 1=w794:dbl)
                    n329 = Multiply(x=w794, y=300) -> (x*y=w792:dbl)
                  }
                  frame True {
                    n330 = local read "v 7"() -> (w801:dbl)
                    n331 = Add(x=w805, y=36) -> (x+y=w806:i32)
                    n332 = Subtract(x=w803, y=w801) -> (x-y=w802:dbl)
                  }
                }
                n333 = case shown="True" w692 {
                  tunnel: [0 w761] -> w690
                  tunnel: w689 -> [_ w760]
                  tunnel: [w747 w757] -> w688
                  tunnel: w687 -> [_ w758]
                  frame False {
                    n334 = call "reset_velocity.vi"() -> ("Numeric"=w750:dbl)  [unwired: 11 in]
                    n335 = local write "v 10"(w750) -> ()
                    n336 = Greater?(x=w750, y=0) -> (0:w752:bool)
                    n337 = case shown="False" w752 {
                      frame False {
                        n338 = local write "Boolean 10"(FALSE) -> ()
                      }
                      frame True {
                        (unwired) 300
                        n339 = local write "Boolean 10"(TRUE) -> ()
                      }
                    }
                    n340 = Random Number (0-1)() -> (number: 0 to 1=w748:dbl)
                    n341 = Multiply(x=w748, y=300) -> (x*y=w747:dbl)
                  }
                  frame True {
                    n342 = Add(x=w760, y=36) -> (x+y=w761:i32)
                    n343 = local read "v 10"() -> (w756:dbl)
                    n344 = Subtract(x=w758, y=w756) -> (x-y=w757:dbl)
                  }
                }
                n345 = case shown="True" w728 {
                  tunnel: [0 w851] -> w726
                  tunnel: w725 -> [_ w850]
                  tunnel: [w837 w847] -> w724
                  tunnel: w723 -> [_ w848]
                  frame False {
                    n346 = call "reset_velocity.vi"() -> ("Numeric"=w840:dbl)  [unwired: 11 in]
                    n347 = local write "v 4"(w840) -> ()
                    n348 = Greater?(x=w840, y=0) -> (0:w842:bool)
                    n349 = case shown="False" w842 {
                      frame False {
                        n350 = local write "Boolean 4"(FALSE) -> ()
                      }
                      frame True {
                        (unwired) 300
                        n351 = local write "Boolean 4"(TRUE) -> ()
                      }
                    }
                    n352 = Random Number (0-1)() -> (number: 0 to 1=w839:dbl)
                    n353 = Multiply(x=w839, y=300) -> (x*y=w837:dbl)
                  }
                  frame True {
                    n354 = Add(x=w850, y=36) -> (x+y=w851:i32)
                    n355 = local read "v 4"() -> (w846:dbl)
                    n356 = Subtract(x=w848, y=w846) -> (x-y=w847:dbl)
                  }
                }
                n357 = case shown="True" w717 {
                  tunnel: [0 w836] -> w719
                  tunnel: w720 -> [_ w835]
                  tunnel: [w822 w832] -> w721
                  tunnel: w722 -> [_ w833]
                  frame False {
                    n358 = call "reset_velocity.vi"() -> ("Numeric"=w825:dbl)  [unwired: 11 in]
                    n359 = local write "v 5"(w825) -> ()
                    n360 = Greater?(x=w825, y=0) -> (0:w827:bool)
                    n361 = case shown="True" w827 {
                      frame False {
                        (unwired) 0
                        n362 = local write "Boolean 5"(FALSE) -> ()
                      }
                      frame True {
                        n363 = local write "Boolean 5"(TRUE) -> ()
                      }
                    }
                    n364 = Random Number (0-1)() -> (number: 0 to 1=w823:dbl)
                    n365 = Multiply(x=w823, y=300) -> (x*y=w822:dbl)
                  }
                  frame True {
                    n366 = local read "v 5"() -> (w831:dbl)
                    n367 = Add(x=w835, y=36) -> (x+y=w836:i32)
                    n368 = Subtract(x=w833, y=w831) -> (x-y=w832:dbl)
                  }
                }
                n369 = case shown="True" w716 {
                  tunnel: [0 w821] -> w714
                  tunnel: w713 -> [_ w820]
                  tunnel: [w807 w817] -> w712
                  tunnel: w711 -> [_ w818]
                  frame False {
                    n370 = call "reset_velocity.vi"() -> ("Numeric"=w810:dbl)  [unwired: 11 in]
                    n371 = local write "v 6"(w810) -> ()
                    n372 = Greater?(x=w810, y=0) -> (0:w812:bool)
                    n373 = case shown="False" w812 {
                      frame False {
                        n374 = local write "Boolean 6"(FALSE) -> ()
                      }
                      frame True {
                        (unwired) 300
                        n375 = local write "Boolean 6"(TRUE) -> ()
                      }
                    }
                    n376 = Random Number (0-1)() -> (number: 0 to 1=w809:dbl)
                    n377 = Multiply(x=w809, y=300) -> (x*y=w807:dbl)
                  }
                  frame True {
                    n378 = Add(x=w820, y=36) -> (x+y=w821:i32)
                    n379 = local read "v 6"() -> (w816:dbl)
                    n380 = Subtract(x=w818, y=w816) -> (x-y=w817:dbl)
                  }
                }
                n381 = case shown="True" w693 {
                  tunnel: [0 w776] -> w695
                  tunnel: w696 -> [_ w775]
                  tunnel: [w762 w772] -> w697
                  tunnel: w698 -> [_ w773]
                  frame False {
                    n382 = call "reset_velocity.vi"() -> ("Numeric"=w765:dbl)  [unwired: 11 in]
                    n383 = local write "v 9"(w765) -> ()
                    n384 = Greater?(x=w765, y=0) -> (0:w767:bool)
                    n385 = case shown="True" w767 {
                      frame False {
                        (unwired) 0
                        n386 = local write "Boolean 9"(FALSE) -> ()
                      }
                      frame True {
                        n387 = local write "Boolean 9"(TRUE) -> ()
                      }
                    }
                    n388 = Random Number (0-1)() -> (number: 0 to 1=w764:dbl)
                    n389 = Multiply(x=w764, y=300) -> (x*y=w762:dbl)
                  }
                  frame True {
                    n390 = Add(x=w775, y=36) -> (x+y=w776:i32)
                    n391 = local read "v 9"() -> (w771:dbl)
                    n392 = Subtract(x=w773, y=w771) -> (x-y=w772:dbl)
                  }
                }
                n393 = case shown="True" w746 {
                  tunnel: [0 w896] -> w744
                  tunnel: w743 -> [_ w895]
                  tunnel: [w882 w892] -> w742
                  tunnel: w741 -> [_ w893]
                  frame False {
                    n394 = call "reset_velocity.vi"() -> ("Numeric"=w885:dbl)  [unwired: 11 in]
                    n395 = local write "v"(w885) -> ()
                    n396 = Greater?(x=w885, y=0) -> (0:w887:bool)
                    n397 = case shown="False" w887 {
                      frame False {
                        n398 = local write "Boolean"(FALSE) -> ()
                      }
                      frame True {
                        n399 = local write "Boolean"(TRUE) -> ()
                      }
                    }
                    n400 = Random Number (0-1)() -> (number: 0 to 1=w884:dbl)
                    n401 = Multiply(x=w884, y=300) -> (x*y=w882:dbl)
                  }
                  frame True {
                    n402 = Add(x=w895, y=36) -> (x+y=w896:i32)
                    n403 = local read "v"() -> (w891:dbl)
                    n404 = Subtract(x=w893, y=w891) -> (x-y=w892:dbl)
                  }
                }
                n405 = call "tree_move.vi"("Left in"=w671, "Top"=w672) -> ("Numeric"=w663:i32, "Left out"=w664:dbl)  [unwired: 8 in]
                n406 = call "tree_move.vi"("Left in"=w676, "Top"=w675) -> ("Numeric"=w667:i32, "Left out"=w668:dbl)  [unwired: 8 in]
                n407 = call "tree_move.vi"("Left in"=w673, "Top"=w674) -> ("Numeric"=w665:i32, "Left out"=w666:dbl)  [unwired: 8 in]
                n408 = call "tree_move.vi"("Left in"=w678, "Top"=w677) -> ("Numeric"=w669:i32, "Left out"=w670:dbl)  [unwired: 8 in]
                n409 = call "tree_move.vi"("Left in"=w681, "Top"=w682) -> ("Numeric"=w680:i32, "Left out"=w679:dbl)  [unwired: 8 in]
                n410 = Increment(x=w684) -> (x+1=w683:i16)
                n411 = property on="Boolean 11" class="Bool (strict)"("Visible"=TRUE) -> ()  [unwired: 2 in, 2 out]
              }
            }
          }
        }
        n412 = property on="tree 5" class="Bool"("Left"=w188, "Top"=w197) -> ()  [unwired: 2 in, 2 out]
        n413 = property on="tree 3" class="Bool"("Left"=w190, "Top"=w199) -> ()  [unwired: 2 in, 2 out]
        n414 = property on="tree 4" class="Bool"("Left"=w189, "Top"=w198) -> ()  [unwired: 2 in, 2 out]
        n415 = property on="tree" class="Bool"("Left"=w192, "Top"=w209) -> ()  [unwired: 2 in, 2 out]
        n416 = property on="tree 2" class="Bool"("Left"=w191, "Top"=w200) -> ()  [unwired: 2 in, 2 out]
        n417 = property on="chicken" class="Bool"("Left"=w215) -> ()  [unwired: 2 in, 2 out]
        n418 = property on="Boolean 2" class="Bool (strict)"("Left"=w241, "Top"=w269) -> ()  [unwired: 2 in, 2 out]
        n419 = property on="Boolean 4" class="Bool (strict)"("Left"=w239, "Top"=w262) -> ()  [unwired: 2 in, 2 out]
        n420 = property on="Boolean 5" class="Bool (strict)"("Left"=w238, "Top"=w260) -> ()  [unwired: 2 in, 2 out]
        n421 = property on="Boolean 3" class="Bool (strict)"("Left"=w240, "Top"=w265) -> ()  [unwired: 2 in, 2 out]
        n422 = property on="Boolean 6" class="Bool (strict)"("Left"=w237, "Top"=w257) -> ()  [unwired: 2 in, 2 out]
        n423 = property on="Boolean 8" class="Bool (strict)"("Left"=w235, "Top"=w250) -> ()  [unwired: 2 in, 2 out]
        n424 = property on="Boolean 7" class="Bool (strict)"("Left"=w236, "Top"=w255) -> ()  [unwired: 2 in, 2 out]
        n425 = property on="Boolean 9" class="Bool (strict)"("Left"=w234, "Top"=w247) -> ()  [unwired: 2 in, 2 out]
        n426 = property on="Boolean 10" class="Bool (strict)"("Left"=w233, "Top"=w244) -> ()  [unwired: 2 in, 2 out]
        n427 = property on="Boolean" class="Bool (strict)"("Left"=w242, "Top"=w268) -> ()  [unwired: 2 in, 2 out]
        n428 = Quotient & Remainder(x=w196, y=w194) -> (x-y*floor(x/y)=w195:i16)  [unwired: 1 out]
        n429 = Subtract(x=w194, y=w195) -> (x-y=w193:i16)
        n430 = case shown="2, 4, 6, 8, 10, Default" w193 {
          tunnel: [10000 w276 w277 w278 w279 w280] -> w186
          tunnel: w192 -> [_ w276 _ _ _ _]
          tunnel: w191 -> [_ _ w277 _ _ _]
          tunnel: w190 -> [_ _ _ w278 _ _]
          tunnel: w189 -> [_ _ _ _ w279 _]
          tunnel: w188 -> [_ _ _ _ _ w280]
          frame 2, 4, 6, 8, 10, Default {
          }
          frame 1 {
          }
          frame 3 {
          }
          frame 5 {
          }
          frame 7 {
          }
          frame 9 {
          }
        }
        n431 = Quotient & Remainder(x=w196, y=i16 10) -> (x-y*floor(x/y)=w229:i16)  [unwired: 1 out]
        n432 = Subtract(x=i16 10, y=w229) -> (x-y=w223:i16)
        n433 = property on="chicken" class="Bool"() -> ("Left"=w187:i32)  [unwired: 2 in, 2 out]
        n434 = case shown="1" w223 {
          tunnel: w242 -> [_ w299 _ _ _ _ _ _ _ _]
          tunnel: w241 -> [_ _ w300 _ _ _ _ _ _ _]
          tunnel: w240 -> [_ _ _ w301 _ _ _ _ _ _]
          tunnel: w239 -> [_ _ _ _ w302 _ _ _ _ _]
          tunnel: w238 -> [_ _ _ _ _ w303 _ _ _ _]
          tunnel: w237 -> [_ _ _ _ _ _ w304 _ _ _]
          tunnel: w236 -> [_ _ _ _ _ _ _ w305 _ _]
          tunnel: w235 -> [_ _ _ _ _ _ _ _ w306 _]
          tunnel: w234 -> [_ _ _ _ _ _ _ _ _ w307]
          tunnel: w233 -> [w298 _ _ _ _ _ _ _ _ _]
          tunnel: [w298 w299 w300 w301 w302 w303 w304 w305 w306 w307] -> w219
          frame 10, Default {
          }
          frame 1 {
          }
          frame 2 {
          }
          frame 3 {
          }
          frame 4 {
          }
          frame 5 {
          }
          frame 6 {
          }
          frame 7 {
          }
          frame 8 {
          }
          frame 9 {
          }
        }
        "car_x" <- w219
        n435 = local write "SCORE"(w196) -> ()
        n436 = Subtract(x=w187, y=w186) -> (x-y=w185:dbl)
        n437 = local read "easy?"() -> (w181:bool)
        n438 = In Range and Coerce(upper limit=24.0, x=w185, lower limit=-24.0) -> (In Range?=w182:bool)  [unwired: 1 out]
        n439 = property on="chicken" class="Bool"() -> ("Left"=w227:i32)  [unwired: 2 in, 2 out]
        n440 = And(x=w182, y=w181) -> (x .and. y?=w178:bool)
        n441 = Quotient & Remainder(x=w223, y=i16 2) -> (x-y*floor(x/y)=w221:i16)  [unwired: 1 out]
        n442 = local read "easy?"() -> (w214:bool)
        n443 = Greater Than 0?(x=w221) -> (x > 0?=w220:bool)
        n444 = And(x=w214, y=w220) -> (x .and. y?=w213:bool)
        n445 = Select(t=10000.0, s=w213, f=w219) -> (s? t:f=w217:dbl)
        n446 = Subtract(x=w227, y=w217) -> (x-y=w226:dbl)
        n447 = In Range and Coerce(upper limit=i16 54 ("lower limit"), x=w226, lower limit=i16 -24) -> (In Range?=w180:bool)  [unwired: 1 out]
        n448 = Or(x=w180, y=w178) -> (x .or. y?=w179:bool)
        n449 = case shown="True" w179 {
          tunnel: w196 -> [_ w295]
          tunnel: [FALSE TRUE] -> w231
          frame False {
          }
          frame True {
            n450 = local read "TOP"() -> (w296:i16)
            n451 = property on="Boolean 12" class="Bool (strict)"("Visible"=TRUE) -> ()  [unwired: 2 in, 2 out]
            n452 = Greater?(x=w295, y=w296) -> (0:w297:bool)
            n453 = Select(t=w295, s=w297, f=w296) -> (s? t:f=w294:i16)
            n454 = local write "TOP"(w294) -> ()
          }
        }
        n455 = case shown="False" w213 {
          frame False {
            n456 = property on="grass 1" class="Bool"("Top"=0) -> ()  [unwired: 2 in, 2 out]
            n457 = property on="grass 2" class="Bool"("Top"=72) -> ()  [unwired: 2 in, 2 out]
            n458 = property on="grass 3" class="Bool"("Top"=144) -> ()  [unwired: 2 in, 2 out]
            n459 = property on="grass 4" class="Bool"("Top"=216) -> ()  [unwired: 2 in, 2 out]
            n460 = property on="grass 5" class="Bool"("Top"=288) -> ()  [unwired: 2 in, 2 out]
          }
          frame True {
            n461 = property on="grass 1" class="Bool"("Top"=36) -> ()  [unwired: 2 in, 2 out]
            n462 = property on="grass 2" class="Bool"("Top"=108) -> ()  [unwired: 2 in, 2 out]
            n463 = property on="grass 3" class="Bool"("Top"=180) -> ()  [unwired: 2 in, 2 out]
            n464 = property on="grass 4" class="Bool"("Top"=252) -> ()  [unwired: 2 in, 2 out]
            n465 = property on="grass 5" class="Bool"("Top"=324) -> ()  [unwired: 2 in, 2 out]
          }
        }
        n466 = Or(x=w231, y="stop") -> (x .or. y?=w230:bool)
      }
      n467 = property on="v" class="DigNum (strict)"("Visible"=w96) -> ()  [unwired: 2 in, 2 out]
      n468 = property on="v 2" class="DigNum (strict)"("Visible"=w96) -> ()  [unwired: 2 in, 2 out]
      n469 = property on="v 3" class="DigNum (strict)"("Visible"=w96) -> ()  [unwired: 2 in, 2 out]
      n470 = property on="v 4" class="DigNum (strict)"("Visible"=w96) -> ()  [unwired: 2 in, 2 out]
      n471 = property on="v 5" class="DigNum (strict)"("Visible"=w96) -> ()  [unwired: 2 in, 2 out]
      n472 = property on="v 6" class="DigNum (strict)"("Visible"=w96) -> ()  [unwired: 2 in, 2 out]
      n473 = property on="v 7" class="DigNum (strict)"("Visible"=w96) -> ()  [unwired: 2 in, 2 out]
      n474 = property on="v 8" class="DigNum (strict)"("Visible"=w96) -> ()  [unwired: 2 in, 2 out]
      n475 = property on="v 9" class="DigNum (strict)"("Visible"=w96) -> ()  [unwired: 2 in, 2 out]
      n476 = property on="v 10" class="DigNum (strict)"("Visible"=w96) -> ()  [unwired: 2 in, 2 out]
      n477 = local write "SCORE"(i16 0 ("score")) -> ()
      n478 = property on="car_x" class="DigNum (strict)"("Visible"=FALSE) -> ()  [unwired: 2 in, 2 out]
    }
  }
  n479 = property on="EASY" class="Bool"("Visible"=w8) -> ()  [unwired: 2 in, 2 out]
  n480 = property on="HARD" class="Bool"("Visible"=w8) -> ()  [unwired: 2 in, 2 out]
  n481 = property on="Boolean 12" class="Bool (strict)"("Visible"=FALSE, "Value"=T1 FALSE ("Boolean 12")) -> ()  [unwired: 2 in, 2 out]
  n482 = property on="Boolean 11" class="Bool (strict)"("Visible"=FALSE) -> ()  [unwired: 2 in, 2 out]
